vi "Configure Calib Factor (Com).vi"(0 "VISA resource name":refnum<visa-resource-name>, 5 "Channel (001)":string="001", 7 "Correct Factor (ON)":bool=TRUE, 9 "Calibration Correction":T1(array[cluster]) {"Sensor Correction Factor" min=-999999 max=999999 step=1; "Instrument Correction Factor" min=-999999 max=999999 step=1; "Uncorrected Value" min=-999999 max=999999 step=1}, 11 "error in (no error)":errorcluster) -> (4 "VISA resource name out":refnum<visa-resource-name>, 6 "Channel":string, 15 "error out":errorcluster)   [LabVIEW 2020, in "Yokogawa GX Series.lvlib"]
doc: "Sets the calibration correction(Correction Factor) for communication channels.\n\nCommand: SCalibUseCom, SCalibCom"
uses:
  <instrlib>/Yokogawa GX Series/Yokogawa GX Series.lvlib
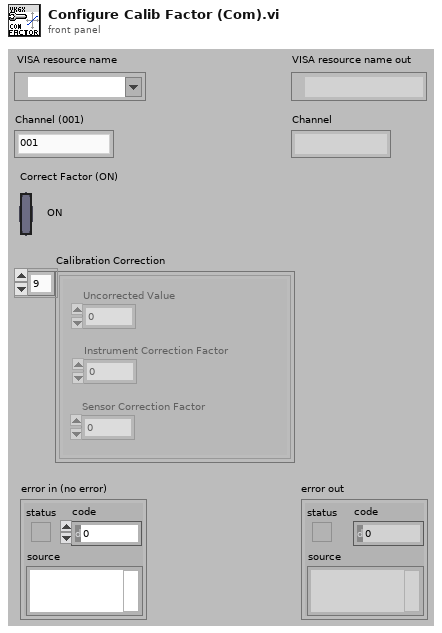
[diagram p1: front panel]
types:
  T1 = cluster{"Uncorrected Value":i32, "Instrument Correction Factor":i32, "Sensor Correction Factor":i32}[]
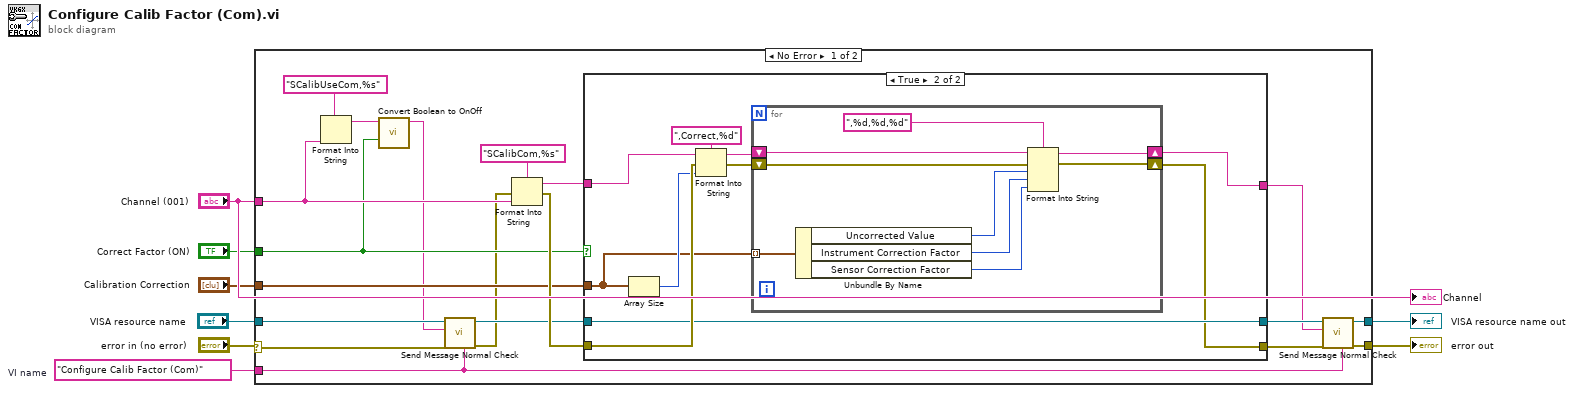
[diagram p0: block diagram]
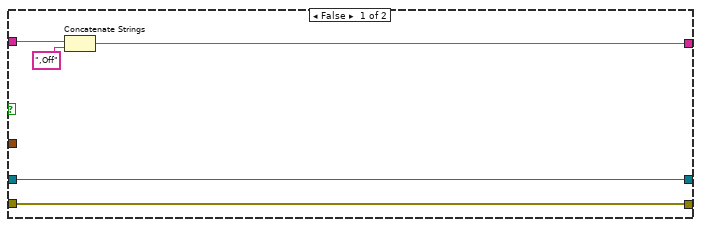
[diagram p2: hidden frame]
diagram:
  w8 = "Configure Calib Factor (Com)"  # VI name
  n1 = case shown="No Error" "error in (no error)" {
    selector: "error in (no error)" -> [w13 w52]
    tunnel: w8 -> [w9 _]
    tunnel: [w27 w53] -> w7
    tunnel: [w26 w52] -> w6
    tunnel: "VISA resource name" -> [w15 w53]
    tunnel: "Channel (001)" -> [w18 _]
    tunnel: "Correct Factor (ON)" -> [w16 _]
    tunnel: "Calibration Correction" -> [w21 _]
    frame No Error {
      n2 = Format Into String(format string="SCalibUseCom,%s", w18) -> (resulting string=w17:string)  [unwired: 2 in, 1 out]
      n3 = call <instrlib>:"Convert Boolean to OnOff.vi"("On/Off"=w16, "Initial String (\"\")"=w17) -> ("Resulting String"=w11:string)  [unwired: 9 in]
      n4 = call <instrlib>:"Send Message Normal Check.vi"("Source (\"\")"=w9, "error in (no error)"=w13, "Send Message (\"\")"=w11, "VISA resource name"=w15) -> ("error out"=w12:errorcluster, "VISA resource name out"=w14:refnum<visa-resource-name>)  [unwired: 2 in, 4 out]
      n5 = Format Into String(format string="SCalibCom,%s", error in=w12, w18) -> (resulting string=w25:string, error out=w24:errorcluster)  [unwired: 1 in]
      n6 = case shown="True" w16 {
        tunnel: w25 -> [w32 w34]
        tunnel: [w30 w38] -> w20
        tunnel: w24 -> [w28 w41]
        tunnel: w14 -> [w29 w37]
        tunnel: [w29 w37] -> w23
        tunnel: [w28 w36] -> w22
        tunnel: w21 -> [_ w33]
        frame False {
          n7 = Concatenate Strings(w32, ",Off") -> (w30:string)
        }
        frame True {
          n8 = Array Size(array=w33) -> (size(s)=w35:i32)
          n9 = Format Into String(format string=",Correct,%d", initial string=w34, error in=w41, w35) -> (resulting string=w40:string, error out=w39:errorcluster)
          n10 = for {
            shift-right: [w48] -> w38
            shift-left: w40 -> [w51]
            shift-right: [w49] -> w36
            shift-left: w39 -> [w50]
            tunnel: w33 -> [w45] mode=indexing
            n11 = Unbundle By Name(w45) -> ("Uncorrected Value"=w46:i32, "Instrument Correction Factor"=w44:i32, "Sensor Correction Factor"=w43:i32)
            n12 = Format Into String(format string=",%d,%d,%d", initial string=w51, error in=w50, w46, w44, w43) -> (resulting string=w48:string, error out=w49:errorcluster)
          }
        }
      }
      n13 = call <instrlib>:"Send Message Normal Check.vi"("Source (\"\")"=w9, "error in (no error)"=w22, "Send Message (\"\")"=w20, "VISA resource name"=w23) -> ("error out"=w26:errorcluster, "VISA resource name out"=w27:refnum<visa-resource-name>)  [unwired: 2 in, 4 out]
    }
    frame Error {
    }
  }
  "error out" <- w6
  "VISA resource name out" <- w7
  "Channel" <- "Channel (001)"
